vi "Read All.vi"(6 "Per Read Size":u64=1024 max=30000, 8 "Error In":errorcluster, 10 "Max Read Size":u64=1024, 11 "SFTP File In":refnum<class "SFTP File.lvclass">) -> (0 "Error Out":errorcluster, 2 "Data":u8[](array[numeric]), 3 "SFTP File Out":refnum<class "SFTP File.lvclass">)   [LabVIEW 2021, in "Field_RnD_Services_LIBSSH2_Toolkit.lvlib" / "SFTP File.lvclass"]
doc: "Reads binary data from a SFTP file represented by this SFTP File object in chunks, or blocks, until the total read size is reached. This VI should be used if the <B>Total Read Size</B> is greater than 30KB because of a hard-coded per-read maximum of 30KB set in the libssh2 shared library."
uses:
  220524-VNA RP FLAT.llb/SFTP File.lvclass
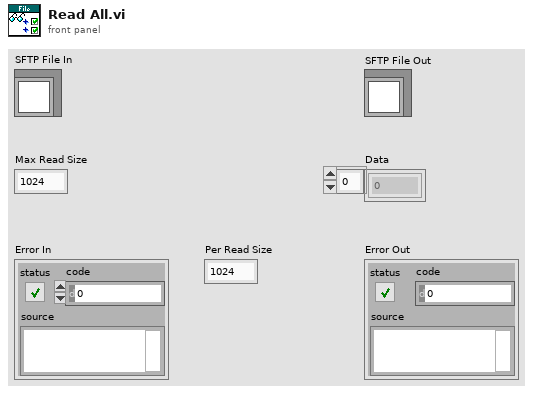
[diagram p1: front panel]
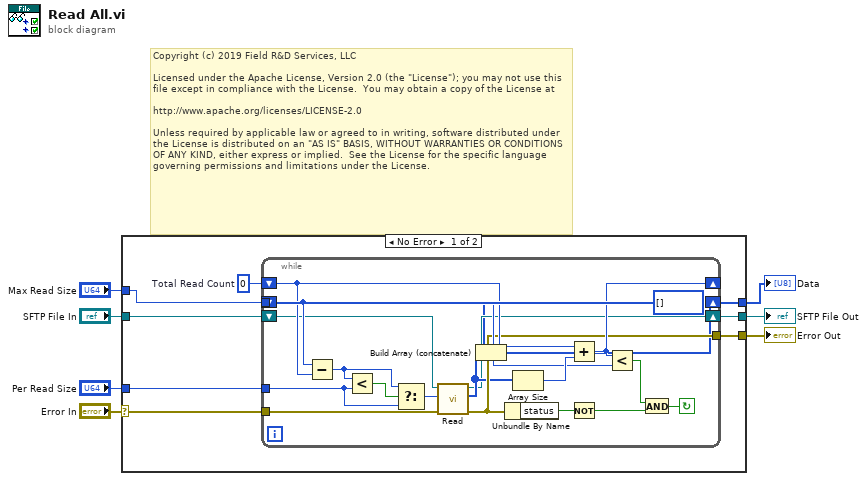
[diagram p0: block diagram]
diagram:
  # "Copyright (c) 2019 Field R&D Services, LLC\n\nLicensed under the Apache License, Version 2.0 (the \"License\"); you may not use this file except in compliance with the License.  You may obtain a copy of the License at\n\nhttp://www.apache.org/licenses/LICENSE-2.0\n\nUnless required by applicable law or agreed to in writing, software distributed under the License is distributed on an \"AS IS\" BASIS, WITHOUT WARRANTIES OR CONDITIONS OF ANY KIND, either express or implied.  See the License for the specific language governing permissions and limitations under the License."
  n1 = case shown="No Error" "Error In" {
    selector: "Error In" -> [w12 w37]
    tunnel: "Max Read Size" -> [w15 _]
    tunnel: "Per Read Size" -> [w14 _]
    tunnel: [w13 _] -> w5
    tunnel: [w11 w37] -> w4
    tunnel: "SFTP File In" -> [w10 w36]
    tunnel: [w9 w36] -> w1
    frame No Error {
      w16 = u64 0  # Total Read Count
      n2 = while {
        shift-right: [w19] -> w9
        shift-left: w10 -> [w20]
        shift-right: [w34] -> _
        shift-left: w16 -> [w32]
        tunnel: w15 -> [w33]
        tunnel: w14 -> [w29]
        tunnel: w12 -> [w24]
        tunnel: [w23] -> w11
        shift-right: [w17] -> w13
        shift-left: u8[] [] ("Data") -> [w18]
        stop <- w25 continue-if-true
        n3 = Subtract(x=w33, y=w32) -> (x-y=w30:u64)
        n4 = Less?(x=w30, y=w29) -> (x < y?=w31:bool)
        n5 = Select(t=w30, s=w31, f=w29) -> (s? t:f=w22:u64)
        n6 = call "Read.vi"("Error In"=w24, "Max Data Length"=w22, "SFTP File In"=w20) -> ("Error Out"=w23:errorcluster, "Data"=w21:u8[], "SFTP File Out"=w19:refnum<class "SFTP File.lvclass">)  [unwired: 6 in]
        n7 = Build Array (concatenate)(w18, w21) -> (w17:u8[])
        n8 = Unbundle By Name(w23) -> ("status"=w28:bool)
        n9 = Array Size(array=w21) -> (size(s)=w35:i32)
        n10 = Add(x=w32, y=w35) -> (x+y=w34:u64)
        n11 = Not(x=w28) -> (.not. x?=w26:bool)
        n12 = Less?(x=w34, y=w33) -> (x < y?=w27:bool)
        n13 = And(x=w27, y=w26) -> (x .and. y?=w25:bool)
      }
    }
    frame Error {
    }
  }
  "Data" <- w5
  "Error Out" <- w4
  "SFTP File Out" <- w1
